vi "fxp32_16-to-int_mul8.vi"(0 "FXP32_16 1":fxp<+/-,32,16>, 1 "FXP32_16 2":fxp<+/-,32,16>, 2 "FXP32_16 3":fxp<+/-,32,16>, 3 "FXP32_16 4":fxp<+/-,32,16>, 4 "FXP32_16 5":fxp<+/-,32,16>, 5 "FXP32_16 6":fxp<+/-,32,16>, 6 "FXP32_16 7":fxp<+/-,32,16>, 7 "FXP32_16 8":fxp<+/-,32,16>) -> (20 "32bit integer 1":i32, 21 "32bit integer 2":i32, 22 "32bit integer 3":i32, 23 "32bit integer 4":i32, 24 "32bit integer 5":i32, 25 "32bit integer 6":i32, 26 "32bit integer 7":i32, 27 "32bit integer 8":i32)   [LabVIEW 2018]
uses:
  <vilib>/rvi/FXPMathLib/FxpInterpret/XNode/nifxpmath_Interpret.xnode
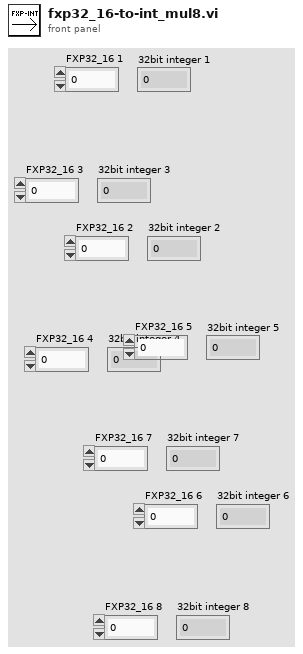
[diagram p1: front panel]
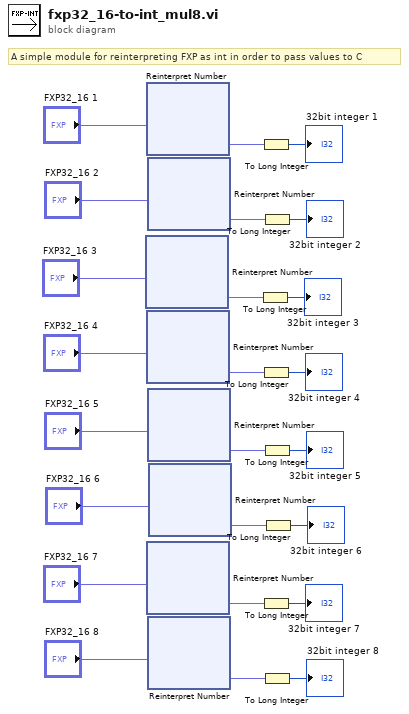
[diagram p0: block diagram]
diagram:
  # "A simple module for reinterpreting FXP as int in order to pass values to C"
  n1 = xnode "Reinterpret Number"("x"="FXP32_16 3") -> ("y"=w17:fxp<+/-,32,32>)
  n2 = xnode "Reinterpret Number"("x"="FXP32_16 1") -> ("y"=w23:fxp<+/-,32,32>)
  n3 = xnode "Reinterpret Number"("x"="FXP32_16 4") -> ("y"=w14:fxp<+/-,32,32>)
  n4 = xnode "Reinterpret Number"("x"="FXP32_16 7") -> ("y"=w5:fxp<+/-,32,32>)
  n5 = xnode "Reinterpret Number"("x"="FXP32_16 2") -> ("y"=w20:fxp<+/-,32,32>)
  n6 = xnode "Reinterpret Number"("x"="FXP32_16 5") -> ("y"=w11:fxp<+/-,32,32>)
  n7 = xnode "Reinterpret Number"("x"="FXP32_16 8") -> ("y"=w2:fxp<+/-,32,32>)
  n8 = xnode "Reinterpret Number"("x"="FXP32_16 6") -> ("y"=w8:fxp<+/-,32,32>)
  n9 = To Long Integer(number=w17) -> (32bit integer=→"32bit integer 3":i32)
  n10 = To Long Integer(number=w23) -> (32bit integer=→"32bit integer 1":i32)
  n11 = To Long Integer(number=w14) -> (32bit integer=→"32bit integer 4":i32)
  n12 = To Long Integer(number=w5) -> (32bit integer=→"32bit integer 7":i32)
  n13 = To Long Integer(number=w20) -> (32bit integer=→"32bit integer 2":i32)
  n14 = To Long Integer(number=w11) -> (32bit integer=→"32bit integer 5":i32)
  n15 = To Long Integer(number=w2) -> (32bit integer=→"32bit integer 8":i32)
  n16 = To Long Integer(number=w8) -> (32bit integer=→"32bit integer 6":i32)
